vi "Expand Variant.vi"(8 "error in (no error)":errorcluster, 9 "Variant":variant, 11 "TwinCAT ADS in":refnum<class "TwinCAT ADS.lvclass">) -> (0 "error out":errorcluster, 1 "Variant Array":variant[](array[variant]), 3 "TwinCAT ADS out":refnum<class "TwinCAT ADS.lvclass">)   [LabVIEW 2018, in "TwinCAT ADS.lvclass"]
uses:
  TwinCAT ADS.lvclass
  <vilib>/Utility/Data Type/NI_Data Type.lvlib
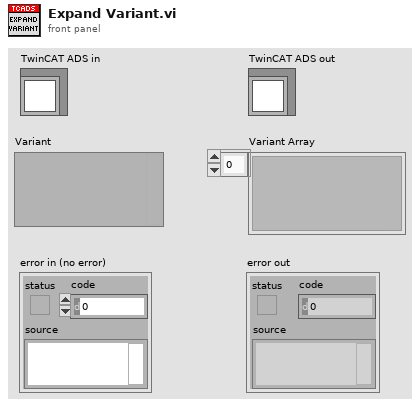
[diagram p1: front panel]
types:
  T1 = typedef "NI_Data Type.lvlib/Data Type.ctl" = enum8{"Invalid Type", "Void", "I8", "I16", "I32", "I64", "U8", "U16", "U32", "U64", "Single Float", "Double Float", "Extended Float", "Single Complex", "Double Complex", "Extended Complex", "Enum U8", "Enum U16", "Enum U32", "Enum U64", "Single Float With Unit", "Double Float With Unit", "Extended Float With Unit", "Single Complex with Unit", "Double Complex with Unit", "Extended Complex with Unit", "Boolean", "String", "Path", "Picture", "Tag", "Array", "Cluster", "Variant", "LV Variant", "Waveform", "Timestamp", "Digital Waveform", "Digital Data", "ExpressData", "Refnum", "External Data", "VI", "Poly VI", "LabVIEW Class Instance", "Fixed Point"}
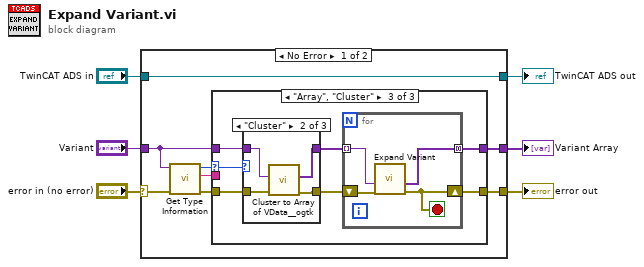
[diagram p0: block diagram]
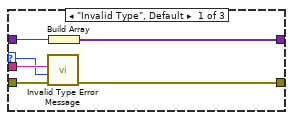
[diagram p2: hidden frame]
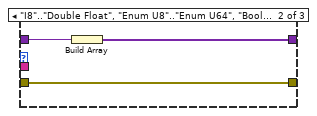
[diagram p3: hidden frame]
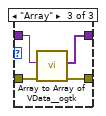
[diagram p5: hidden frame]
diagram:
  n1 = case shown="No Error" "error in (no error)" {
    selector: "error in (no error)" -> [w14 w45]
    tunnel: [w8 w45] -> w5
    tunnel: [w7 w44] -> w3
    tunnel: "TwinCAT ADS in" -> [w7 w44]
    tunnel: "Variant" -> [w12 _]
    tunnel: [w9 _] -> w1
    frame No Error {
      n2 = call <vilib>:"Get Type Information.vi"("error in (no error)"=w14, "Variant"=w12) -> ("error out"=w11:errorcluster, "Name"=w10:string, "Type"=w13:T1)  [unwired: 5 in, 2 out]
      n3 = case shown="\"Array\", \"Cluster\"" w13 {
        selector: w13 -> [w18 _ w25]
        tunnel: w12 -> [w16 w22 w29]
        tunnel: w11 -> [w20 w21 w30]
        tunnel: w10 -> [w19 _ _]
        tunnel: [w17 w21 w24] -> w8
        tunnel: [w15 w23 w26] -> w9
        frame "Invalid Type", Default {
          n4 = call "Invalid Type Error Message.vi"("error in (no error)"=w20, "Type"=w18, "Name"=w19) -> ("error out"=w17:errorcluster)  [unwired: 7 in, 1 out]
          n5 = Build Array(w16) -> (w15:variant[])
        }
        frame "I8".."Double Float", "Enum U8".."Enum U64", "Boolean", "String" {
          n6 = Build Array(w22) -> (w23:variant[])
        }
        frame "Array", "Cluster" {
          n7 = case shown="\"Cluster\"" w25 {
            tunnel: w30 -> [w31 w35 w39]
            tunnel: w29 -> [_ w34 w37]
            tunnel: [w31 w33 w38] -> w28
            tunnel: [_ w32 w36] -> w27
            frame "Invalid Type", Default {
            }
            frame "Cluster" {
              n8 = call <userlib>:"Cluster to Array of VData__ogtk.vi"("error in (no error)"=w35, "Cluster"=w34) -> ("error out"=w33:errorcluster, "Array of VData"=w32:variant[])  [unwired: 8 in]
            }
            frame "Array" {
              n9 = call <userlib>:"Array to Array of VData__ogtk.vi"("error in (no error)"=w39, "MultiD Array"=w37) -> ("error out"=w38:errorcluster, "1D Array of Variants"=w36:variant[])  [unwired: 8 in]
            }
          }
          n10 = for {
            tunnel: w27 -> [w42] mode=indexing
            tunnel: [w41] -> w26 mode=concatenating
            shift-right: [w40] -> w24
            shift-left: w28 -> [w43]
            stop <- w40 stop-if-true
            n11 = call "Expand Variant.vi"("error in (no error)"=w43, "Variant"=w42) -> ("error out"=w40:errorcluster, "Variant Array"=w41:variant[])  [unwired: 7 in, 1 out]
          }
        }
      }
    }
    frame Error {
    }
  }
  "error out" <- w5
  "TwinCAT ADS out" <- w3
  "Variant Array" <- w1
